vi "ImportFilter.vi"(8 "error in (no error)":errorcluster, 10 "Clust Refnum":refnum<vi>, 11 "Database in":refnum<class "Database.lvclass">) -> (0 "error out":errorcluster, 2 "Clust Refnum 2":refnum<vi>, 3 "Database out":refnum<class "Database.lvclass">)   [LabVIEW 2014, in "Database.lvclass"]
uses:
  Database.lvclass
  Database.lvclass/Database.ctl
  <vilib>/addons/database/NI_Database_API.lvlib
panel:
  in  "session__p_m_t_filter_set":T1
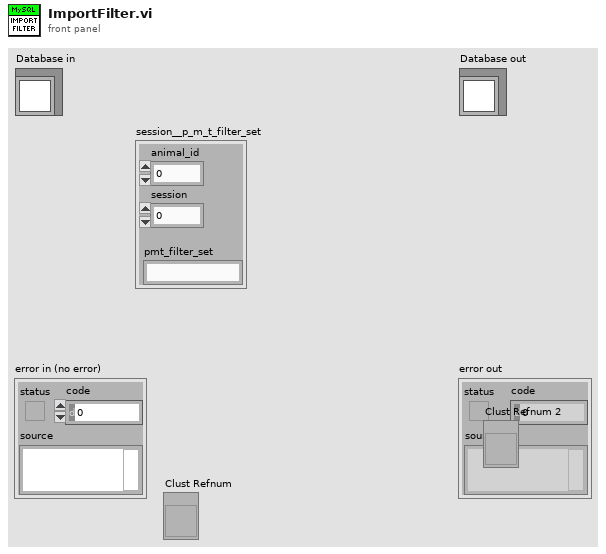
[diagram p1: front panel]
types:
  T1 = cluster{"animal_id":dbl, "session":dbl, "pmt_filter_set":string}
  T2 = typedef "NI_Database_API.lvlib/Conn ObjectReference.ctl" = refnum<k1>
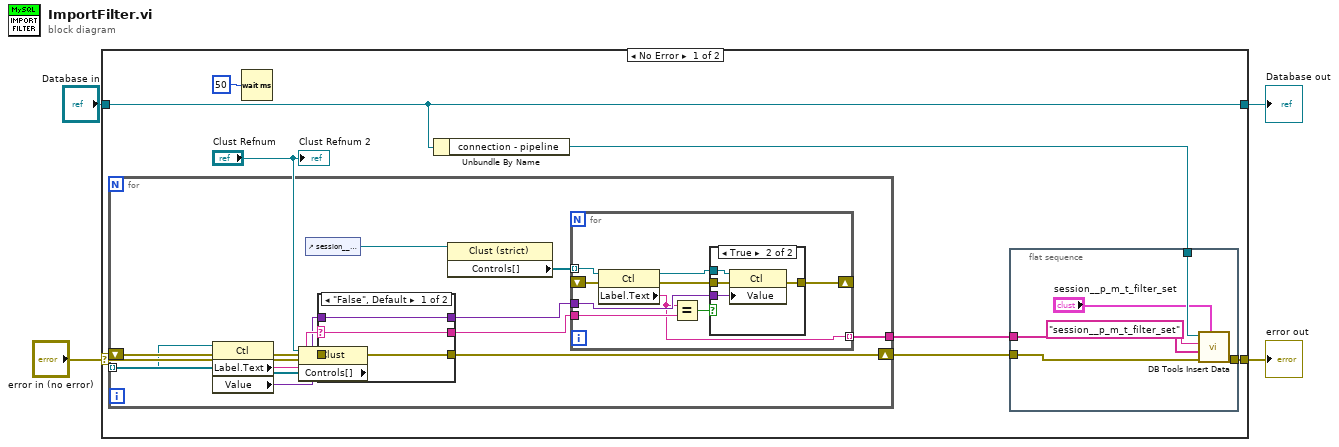
[diagram p0: block diagram]
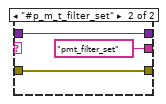
[diagram p3: hidden frame]
diagram:
  n1 = case shown="No Error" "error in (no error)" {
    selector: "error in (no error)" -> [w8 w53]
    tunnel: [w6 w53] -> w3
    tunnel: [w7 w52] -> w1
    tunnel: "Database in" -> [w7 w52]
    frame No Error {
      n2 = Wait (ms)(milliseconds to wait=u32 50) -> ()  [unwired: 1 out]
      n3 = property class="Clust"(reference="Clust Refnum", error in=w8) -> (error out=w13:errorcluster, "Controls[]"=w14:refnum<vi>[])  [unwired: 1 out]
      n4 = for {
        tunnel: w14 -> [w31] mode=indexing
        shift-right: [w21] -> w10
        shift-left: w13 -> [w30]
        tunnel: [w23] -> w12
        n5 = property class="Ctl"(reference=w31, error in=w30) -> (error out=w28:errorcluster, "Label.Text"=w29:string, "Value"=w27:variant)  [unwired: 1 out]
        n6 = control-ref of="session__p_m_t_filter_set"() -> (w22:refnum<vi>)
        n7 = case shown="\"False\", Default" w29 {
          selector: w29 -> [w48 _]
          tunnel: [w48 "pmt_filter_set"] -> w24
          tunnel: w28 -> [w47 w50]
          tunnel: [w47 w50] -> w21
          tunnel: w27 -> [w46 w49]
          tunnel: [w46 w49] -> w25
          frame "False", Default {
          }
          frame "#p_m_t_filter_set" {
          }
        }
        n8 = property class="Clust (strict)"(reference=w22) -> ("Controls[]"=w26:refnum<vi>[])  [unwired: 1 in, 2 out]
        n9 = for {
          tunnel: w24 -> [w40]
          tunnel: w25 -> [w37]
          tunnel: w26 -> [w39] mode=indexing
          tunnel: [w35] -> w23 mode=indexing
          shift-right: [w32] -> _
          shift-left: _ -> [w34]
          n10 = property class="Ctl"(reference=w39, error in=w34) -> (reference out=w38:refnum<vi>, error out=w33:errorcluster, "Label.Text"=w35:string)
          n11 = Equal?(x=w35, y=w40) -> (x = y?=w36:bool)
          n12 = case shown="True" w36 {
            tunnel: w38 -> [_ w45]
            tunnel: w37 -> [_ w44]
            tunnel: w33 -> [w41 w43]
            tunnel: [w41 w42] -> w32
            frame False {
            }
            frame True {
              n13 = property class="Ctl"(reference=w45, error in=w43, "Value"=w44) -> (error out=w42:errorcluster)  [unwired: 1 out]
            }
          }
        }
      }
      n14 = Unbundle By Name(w7) -> ("connection - pipeline"=w9:T2)
      n15 = flat-sequence {
        tunnel: w12 -> [w20]
        tunnel: w10 -> [w18]
        tunnel: w9 -> [w17]
        tunnel: [w16] -> w6
        frame #0 {
          n16 = call <vilib>:"DB Tools Insert Data.vi"("data"="session__p_m_t_filter_set", "error in (no error)"=w18, "columns"=w20, "table"="session__p_m_t_filter_set" ("session"), "connection reference"=w17) -> ("error out"=w16:errorcluster)  [unwired: 5 in, 1 out]
        }
      }
      "Clust Refnum 2" <- "Clust Refnum"
    }
    frame Error {
    }
  }
  "error out" <- w3
  "Database out" <- w1
